vi "CSM_Item_OnPopupMenu.vi"(11 "Object":T1) -> ()   [LabVIEW 2014]
uses:
  <resource>/Framework/Providers/API/ItemRef.ctl
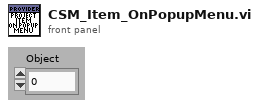
[diagram p1: front panel]
types:
  T1 = typedef "ItemRef.ctl" = u64
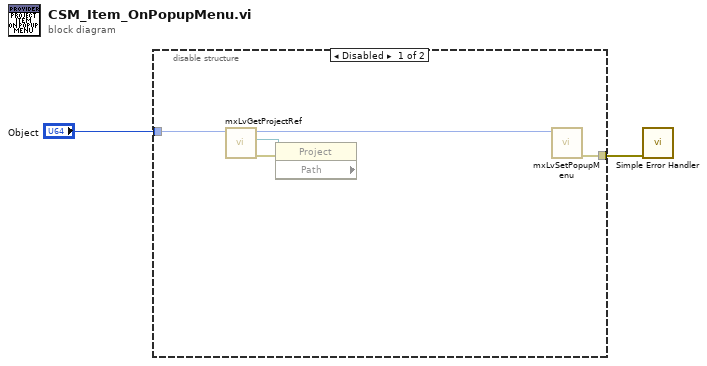
[diagram p0: block diagram]
diagram:
  n1 = disable-structure shown="Disabled" {
    disable-tunnel: [w7 _] -> w2
    disable-tunnel: "Object" -> [w4 _]
    frame Disabled {
      n2 = call <resource>:"mxLvGetProjectRef.vi"("Item"=w4) -> ("error out"=w6:errorcluster, "Project Refnum"=w5:refnum<vi>, "Item"=w3:T1)  [unwired: 8 in]
      n3 = property class="Project" props=["Path"](reference=w5, error in=w6) -> ()  [unwired: 3 out]
      n4 = call <resource>:"mxLvSetPopupMenu.vi"("Item"=w3) -> ("error out"=w7:errorcluster)  [unwired: 9 in, 1 out]
    }
    frame Enabled {
    }
  }
  n5 = call <vilib>:"Simple Error Handler.vi"("error in (no error)"=w2) -> ()  [unwired: 4 in, 5 out]
